vi "bin_temp.vi"() -> ()   [LabVIEW 2013]
panel:
  out "marker":dbl[](array[numeric])
  out "frame_mk":dbl[](array[numeric])
  out "taustream":dbl[][](array[numeric])
  out "matlab error":errorcluster
  in  "data":dbl[](array[numeric]) format="%#.6f"
  in  "extra":dbl
  in  "yPixels":dbl
  in  "xPixels":dbl
  in  "sAOxy":dbl
  in  "sample rate":dbl
  in  "frame time":dbl
  in  "resolution":dbl
  in  "sync time":dbl
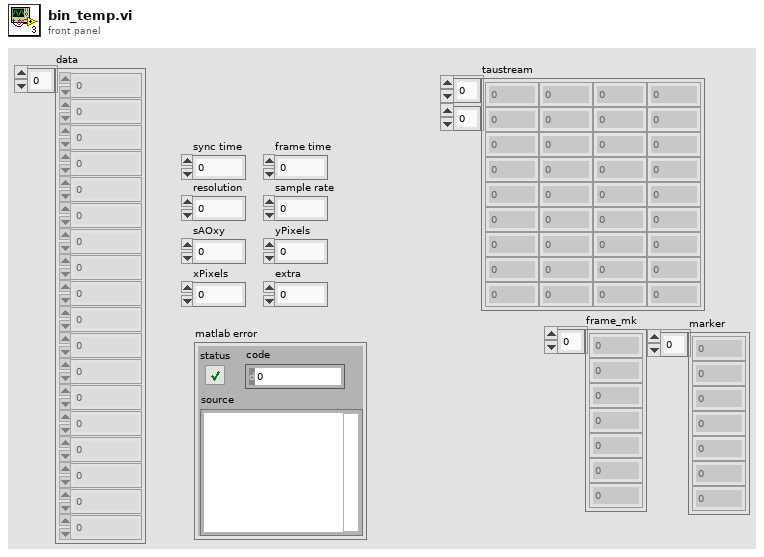
[diagram p1: front panel]
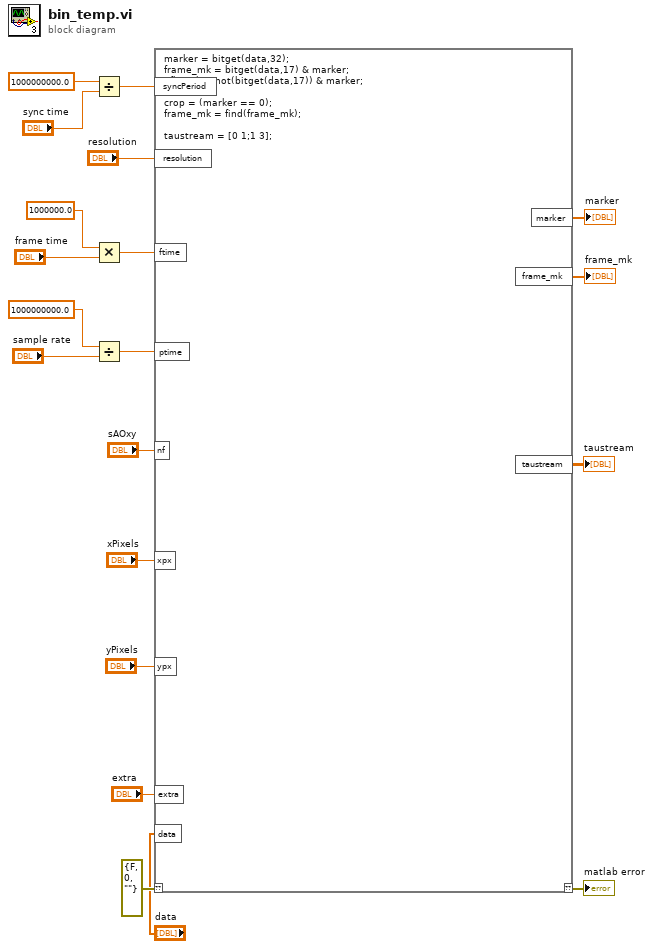
[diagram p0: block diagram]
diagram:
  n1 = Divide(x=1000000000.0, y="sync time") -> (x/y=w13:dbl)
  n2 = Multiply(x=1000000.0, y="frame time") -> (x*y=w11:dbl)
  n3 = Divide(x=1000000000.0, y="sample rate") -> (x/y=w7:dbl)
  n4 = script code="marker = bitget(data,32);\nframe_mk = bitget(data,17) & marker;\noflo_mk = not(bitget(data,17)) & marker;\n\ncrop = (marker == 0);\nframe_mk = find(frame_mk);\n\ntaustream = [0 1;1 3];"("??"=errorcluster {"status"=FALSE, "code"=0, "source"=""} ("error in"), "syncPeriod"=w13, "resolution"="resolution", "ftime"=w11, "ptime"=w7, "nf"="sAOxy", "xpx"="xPixels", "ypx"="yPixels", "extra"="extra", "data"="data") -> ("??"=→"matlab error":errorcluster, "taustream"=→"taustream":dbl[][], "frame_mk"=→"frame_mk":dbl[], "marker"=→"marker":dbl[])
